vi "DB_Insert Data.vi"(7 "data":variant, 8 "error in (no error)":errorcluster, 9 "columns":string[](array[string]), 10 "table":string, 11 "connection reference":T1) -> (0 "error out":errorcluster)   [LabVIEW 2017]
uses:
  <vilib>/addons/database/Connection.llb/Conn ObjectReference.ctl
  <vilib>/addons/database/NI_Database_API.lvlib
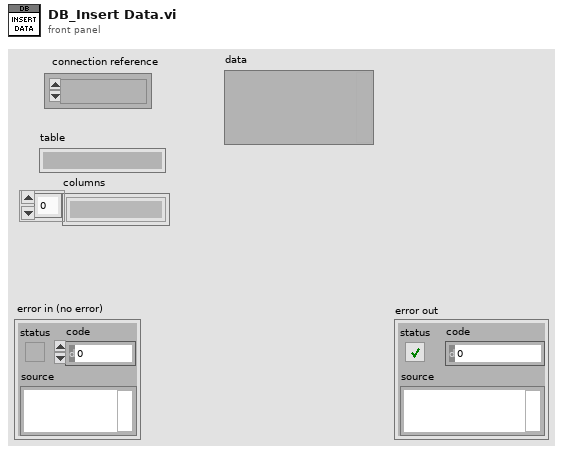
[diagram p1: front panel]
types:
  T1 = typedef "NI_Database_API.lvlib/Conn ObjectReference.ctl" = refnum<k1>
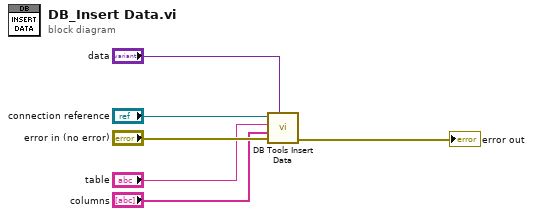
[diagram p0: block diagram]
diagram:
  n1 = call <vilib>:"DB Tools Insert Data.vi"("data"="data", "error in (no error)"="error in (no error)", "columns"="columns", "table"="table", "connection reference"="connection reference") -> ("error out"=→"error out":errorcluster)  [unwired: 5 in, 1 out]
